vi "FTW-JSON-Core-LibraryReturnValue.vi"(0 "error in":errorcluster, 7 "Return Code":i64) -> (4 "error out":errorcluster)   [LabVIEW 2015]
panel:
  # "Inputs"
  # "Outputs"
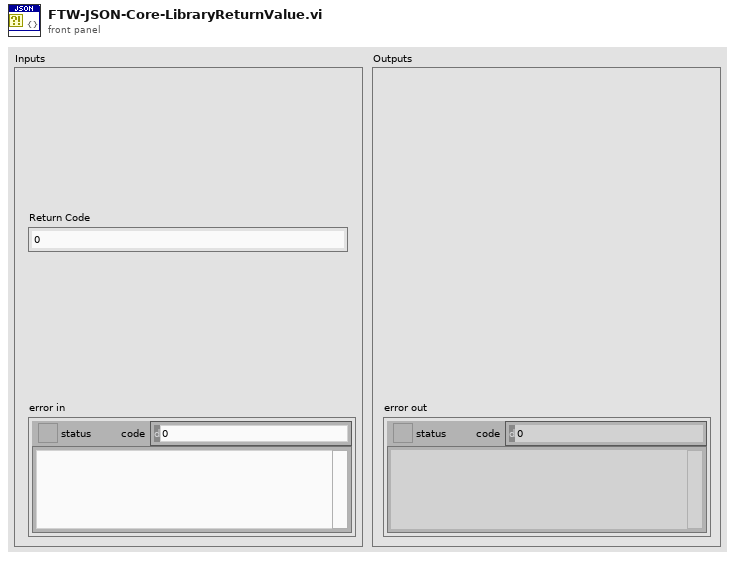
[diagram p1: front panel]
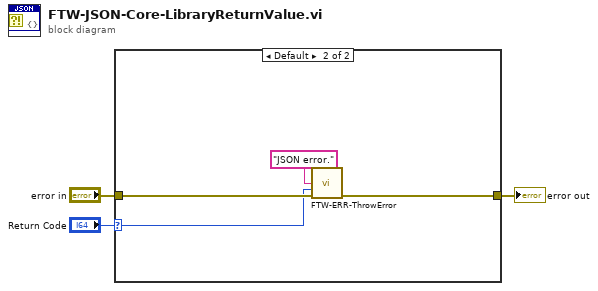
[diagram p0: block diagram]
diagram:
  n1 = case shown="Default" "Return Code" {
    selector: "Return Code" -> [_ w5]
    tunnel: "error in" -> [w4 w7]
    tunnel: [w4 w8] -> w2
    frame 0 {
    }
    frame Default {
      n2 = call "FTW-ERR-ThrowError.vi"("Error Message"="JSON error.", "Error Code"=w5, "error in"=w7) -> ("error out"=w8:errorcluster)  [unwired: 12 in]
    }
  }
  "error out" <- w2
